vi "RNN_Backward_Pass_demo.vi"() -> ()   [LabVIEW 2014]
uses:
  <vilib>/Analysis/Matrix/Datatypes/RealMatrix.ctl
  <vilib>/Analysis/baseanly.llb/A x Vector.vi
  <vilib>/Analysis/Matrix/Numeric/Conversions/Array To Matrix - RA.vi
  <vilib>/Analysis/Matrix/Numeric/Add/Add - RM,RM.vi
  <vilib>/Analysis/NI_AALBase.lvlib
  <vilib>/Analysis/Matrix/NI_Matrix.lvlib
panel:
  in  "params 2":T2
  in  "dParams":T3
  out "dParams":T3
  in  "dby":T1
  in  "dbh":T1
  in  "dWhy":T1
  in  "dWhh":T1
  in  "dWxh":T1
  out "dby":T1
  out "dbh":T1
  out "dWhy":T1
  out "dWhh":T1
  out "dWxh":T1
  in  "ps 2":dbl[][][](array[numeric])
  out "Random Array (1D)":dbl[](array[numeric])
  in  "Length":i32
  out "Array (2D)":dbl[][](array[numeric])
  in  "Matrix":T1
  in  "Matrix 2":T1
  out "Array (1D)":dbl[](array[numeric])
  in  "targets":i64[](array[numeric])
  in  "params":T2
  in  "hs":dbl[][][](array[numeric])
  in  "ps":dbl[][][](array[numeric])
  in  "xs":dbl[][][](array[numeric])
  out "length":i32
  in  "inputs":i32[](array[numeric])
  out "t":i32
  out "t (reversed)":i32
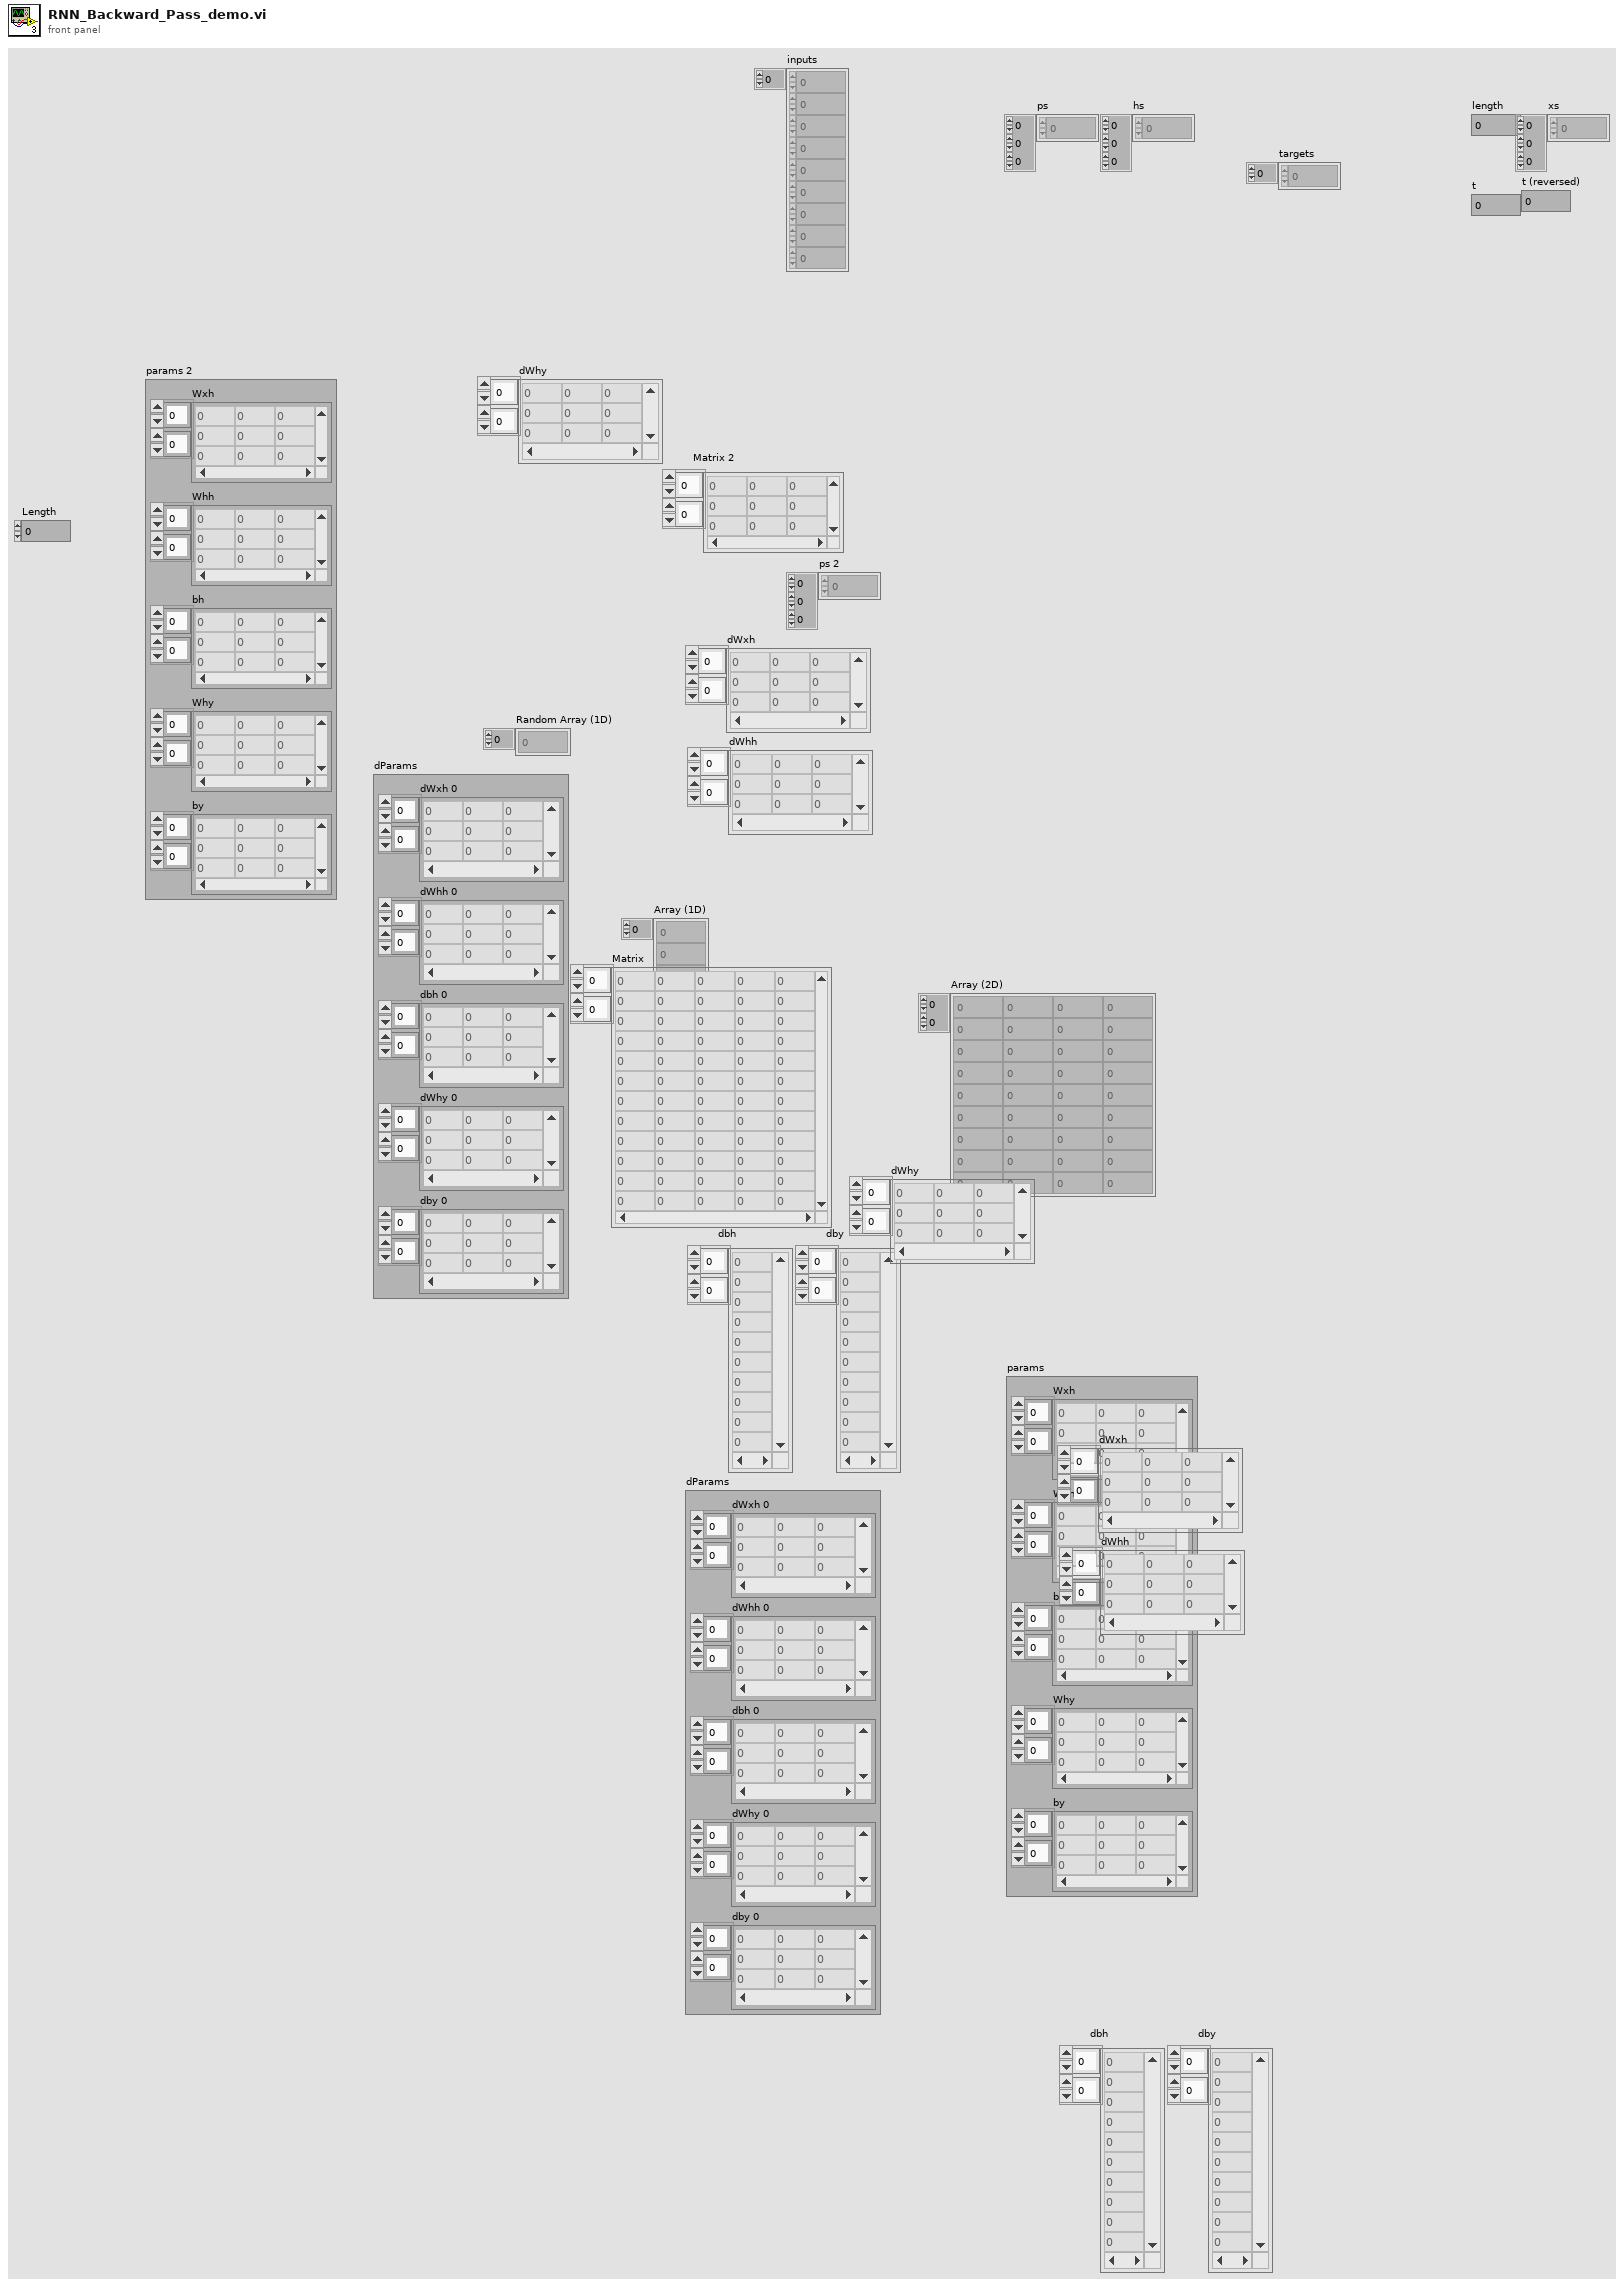
[diagram p1: front panel]
types:
  T1 = typedef "NI_Matrix.lvlib/RealMatrix.ctl" = dbl[][]
  T2 = cluster{"Wxh":T1, "Whh":T1, "bh":T1, "Why":T1, "by":T1}
  T3 = cluster{"dWxh 0":T1, "dWhh 0":T1, "dbh 0":T1, "dWhy 0":T1, "dby 0":T1}
  T4 = cluster{"A + B":T1, "A + B":T1, "Real Matrix (Column Vector)":T1, "A + B":T1, "Real Matrix (Column Vector)":T1}
  T5 = cluster{"dWxh":T1, "dWhh":T1, "dbh":T1, "dWhy":T1, "dby":T1}
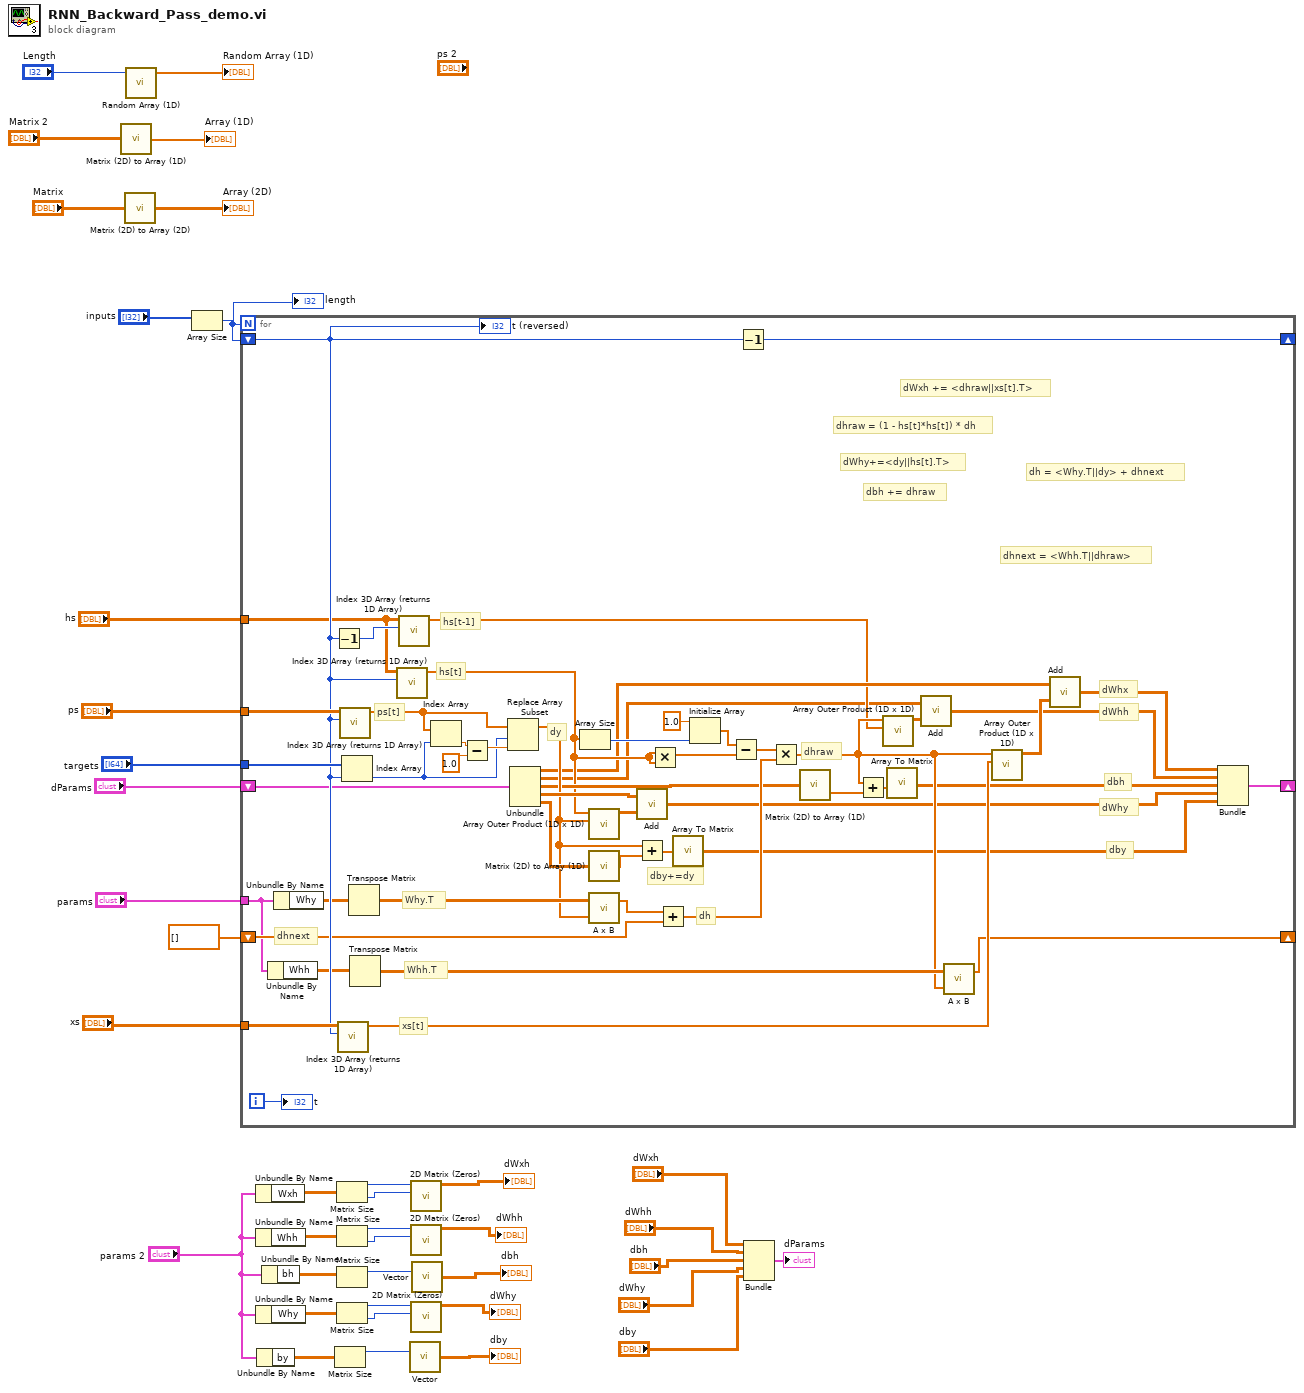
[diagram p0: block diagram]
diagram:
  n1 = call "Matrix (2D) to Array (1D).vi"("Matrix (2D)"="Matrix 2") -> ("Array (1D)"=→"Array (1D)":dbl[])  [unwired: 4 in]
  n2 = call "Matrix (2D) to Array (2D).vi"("Matrix"="Matrix") -> ("Array"=→"Array (2D)":dbl[][])  [unwired: 4 in]
  n3 = call "Random Array (1D).vi"("Length"="Length") -> ("Random Array (1D)"=→"Random Array (1D)":dbl[])  [unwired: 4 in]
  n4 = Array Size(array="inputs") -> (size(s)=w37:i32)
  "length" <- w37
  n5 = for {
    N: w37 -> [_]
    shift-right: [w44] -> _
    shift-left: "dParams" -> [w76]
    tunnel: "xs" -> [w88]
    tunnel: "hs" -> [w84]
    tunnel: "ps" -> [w87]
    tunnel: "params" -> [w42]
    shift-right: [w90] -> _
    shift-left: w37 -> [w86]
    tunnel: "targets" -> [w89]
    shift-right: [w55] -> _
    shift-left: dbl[] [] ("1D array") -> [w70]
    i -> [w91]
    # "dby"
    # "dWhy"
    # "dhnext = <Whh.T||dhraw>"
    # "Whh.T"
    # "dWxh += <dhraw||xs[t].T>"
    # "dWhh"
    # "dWhx"
    # "dy"
    # "dbh"
    # "dhraw"
    # "dbh += dhraw"
    # "dhraw = (1 - hs[t]*hs[t]) * dh"
    # "dh = <Why.T||dy> + dhnext"
    # "dh"
    # "dhnext"
    # "Why.T"
    # "dWhy+=<dy||hs[t].T>"
    # "dby+=dy"
    # "hs[t-1]"
    # "hs[t]"
    # "xs[t]"
    # "ps[t]"
    n6 = Unbundle By Name(w42) -> ("Whh"=w43:T1)
    n7 = Unbundle By Name(w42) -> ("Why"=w41:T1)
    n8 = Decrement(x=w86) -> (x-1=w85:i32)
    n9 = call "Index 3D Array (returns 1D Array).vi"("index"=w86, "3D array"=w88) -> ("1D array"=w59:dbl[])  [unwired: 9 in]
    n10 = call "Index 3D Array (returns 1D Array).vi"("index"=w86, "3D array"=w87) -> ("1D array"=w81:dbl[])  [unwired: 9 in]
    n11 = Index Array(array=w89, index=w86) -> (element=w79:i64)
    n12 = Transpose Matrix(1:w41) -> (0:w72:T1)
    n13 = Transpose Matrix(1:w43) -> (0:w56:T1)
    n14 = call "Index 3D Array (returns 1D Array).vi"("index"=w86, "3D array"=w84) -> ("1D array"=w60:dbl[])  [unwired: 9 in]
    n15 = call "Index 3D Array (returns 1D Array).vi"("index"=w85, "3D array"=w84) -> ("1D array"=w53:dbl[])  [unwired: 9 in]
    n16 = Index Array(array=w81, index=w79) -> (element=w83:dbl)
    n17 = Subtract(x=w83, y=1.0) -> (x-y=w80:dbl)
    n18 = Replace Array Subset(array=w81, new element=w80, index=w79) -> (w65:dbl[])
    n19 = Unbundle(w76) -> ("dWxh 0"=w58:T1, "dWhh 0"=w52:T1, "dbh 0"=w61:T1, "dWhy 0"=w74:T1, "dby 0"=w75:T1)
    n20 = Array Size(array=w60) -> (size(s)=w69:i32)
    n21 = call "Array Outer Product (1D x 1D).vi"("array b"=w65, "array a"=w60) -> ("a X b"=w73:dbl[][])  [unwired: 9 in]
    n22 = call "Matrix (2D) to Array (1D).vi"("Matrix (2D)"=w75) -> ("Array (1D)"=w77:dbl[])  [unwired: 4 in]
    n23 = call-poly <vilib>:"A x B.vi"("Vector"=w65, "A"=w72) -> ("A x Vector"=w71:dbl[])  [unwired: 1 out]
    n24 = call-poly <vilib>:"Add.vi"("Real Matrix B"=w73, "Real Matrix A"=w74) -> ("A + B"=w46:T1)
    n25 = Add(x=w65, y=w77) -> (x+y=w78:dbl[])
    n26 = Multiply(x=w60, y=w60) -> (x*y=w66:dbl[])
    n27 = Add ("Add.vi")(x=w71, y=w70) -> (x+y=w64:dbl[])
    n28 = call-poly <vilib>:"Array To Matrix.vi"("Real 1D Array"=w78) -> ("Real Matrix (Column Vector)"=w45:T1)
    n29 = Initialize Array(1.0 ("element"), w69) -> (w67:dbl[])
    n30 = Subtract(x=w67, y=w66) -> (x-y=w63:dbl[])
    n31 = Decrement(x=w86) -> (x-1=w90:i32)
    n32 = Multiply(x=w63, y=w64) -> (x*y=w54:dbl[])
    n33 = call "Matrix (2D) to Array (1D).vi"("Matrix (2D)"=w61) -> ("Array (1D)"=w62:dbl[])  [unwired: 4 in]
    n34 = Add ("Add.vi")(x=w54, y=w62) -> (x+y=w48:dbl[])
    n35 = call "Array Outer Product (1D x 1D).vi"("array b"=w53, "array a"=w54) -> ("a X b"=w51:dbl[][])  [unwired: 9 in]
    n36 = call-poly <vilib>:"Array To Matrix.vi"("Real 1D Array"=w48) -> ("Real Matrix (Column Vector)"=w47:T1)
    n37 = call-poly <vilib>:"Add.vi"("Real Matrix B"=w51, "Real Matrix A"=w52) -> ("A + B"=w49:T1)
    n38 = call-poly <vilib>:"A x B.vi"("Vector"=w54, "A"=w56) -> ("A x Vector"=w55:dbl[])  [unwired: 1 out]
    n39 = call "Array Outer Product (1D x 1D).vi"("array b"=w59, "array a"=w54) -> ("a X b"=w57:dbl[][])  [unwired: 9 in]
    n40 = call-poly <vilib>:"Add.vi"("Real Matrix B"=w57, "Real Matrix A"=w58) -> ("A + B"=w50:T1)
    n41 = Bundle("A + B"=w50, "A + B"=w49, "Real Matrix (Column Vector)"=w47, "A + B"=w46, "Real Matrix (Column Vector)"=w45) -> (w44:T4)  [unwired: 1 in]
    "t" <- w91
    "t (reversed)" <- w86
  }
  n42 = Unbundle By Name("params 2") -> ("Wxh"=w28:T1)
  n43 = Unbundle By Name("params 2") -> ("Whh"=w25:T1)
  n44 = Unbundle By Name("params 2") -> ("Why"=w22:T1)
  n45 = Unbundle By Name("params 2") -> ("by"=w15:T1)
  n46 = Unbundle By Name("params 2") -> ("bh"=w18:T1)
  n47 = Matrix Size(0:w15) -> (1:w16:i32)  [unwired: 1 out]
  n48 = Matrix Size(0:w28) -> (1:w26:i32, 2:w27:i32)
  n49 = Matrix Size(0:w25) -> (1:w23:i32, 2:w24:i32)
  n50 = Matrix Size(0:w18) -> (1:w17:i32)  [unwired: 1 out]
  n51 = Matrix Size(0:w22) -> (1:w20:i32, 2:w21:i32)
  n52 = call "Vector.vi"("length"=w16) -> ("Real Matrix (Column Vector)"=→"dby":T1)  [unwired: 1 in]
  n53 = call "2D Matrix (Zeros).vi"("nCols (1)"=w27, "nRows"=w26) -> ("Real Matrix"=→"dWxh":T1)  [unwired: 9 in]
  n54 = call "2D Matrix (Zeros).vi"("nCols (1)"=w24, "nRows"=w23) -> ("Real Matrix"=→"dWhh":T1)  [unwired: 9 in]
  n55 = call "2D Matrix (Zeros).vi"("nCols (1)"=w21, "nRows"=w20) -> ("Real Matrix"=→"dWhy":T1)  [unwired: 9 in]
  n56 = call "Vector.vi"("length"=w17) -> ("Real Matrix (Column Vector)"=→"dbh":T1)  [unwired: 1 in]
  n57 = Bundle("dWxh"="dWxh", "dWhh"="dWhh", "dbh"="dbh", "dWhy"="dWhy", "dby"="dby") -> (→"dParams":T5)  [unwired: 1 in]
